vi "Filter Event Data.vi"(8 "error in (no error)":errorcluster, 10 "EventFilter Reference":T1, 11 "ControlDragStartingMsg In":refnum<class "ControlDragStartingMsg.lvclass">) -> (0 "error out":errorcluster, 2 "Discard?":bool, 3 "ControlDragStartingMsg Out":refnum<class "ControlDragStartingMsg.lvclass">)   [LabVIEW 2019, in "ActorEvents.lvlib" / "ControlDragStartingMsg.lvclass"]
uses:
  <vilib>/gpm_packages/@cs/mva-viewable/Source/ActorEvents/IEventAggregator Messages/ControlDragStartingMsg/ControlDragStartingMsg.lvclass
  <vilib>/gpm_packages/@cs/mva-viewable/Source/ActorEvents/IEventFilter/EventFilter Reference.ctl
  <vilib>/gpm_packages/@cs/mva-viewable/Source/ActorEvents/IEventFilter/IEventFilter.lvclass
  <vilib>/gpm_packages/@cs/mva-viewable/Source/ActorEvents/IEventAggregator Messages/ControlDragStartingMsg/ControlDragStartingMsg.lvclass/ControlDragStartingMsg.ctl
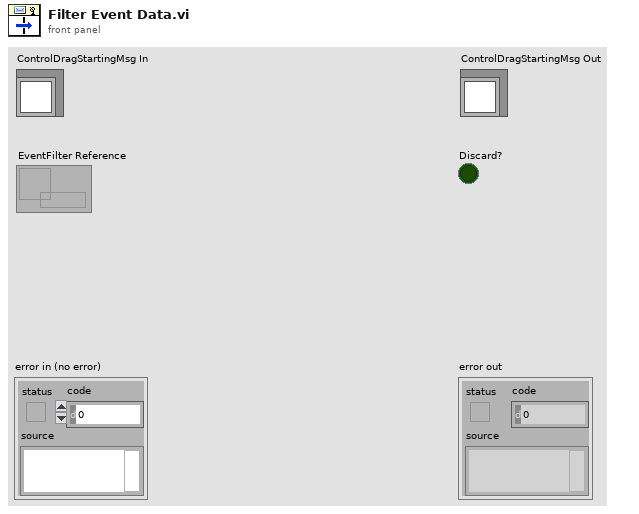
[diagram p1: front panel]
types:
  T1 = typedef "ActorEvents.lvlib/IEventFilter.lvclass/EventFilter Reference.ctl" = refnum<data-value>
  T2 = cluster{"Data":cluster{"data name":string, "drag data":variant}[], "Drag Mode":enum32{"copy or move", "copy only", "move only"}}
  T3 = cluster{"data name":string, "drag data":variant}[]
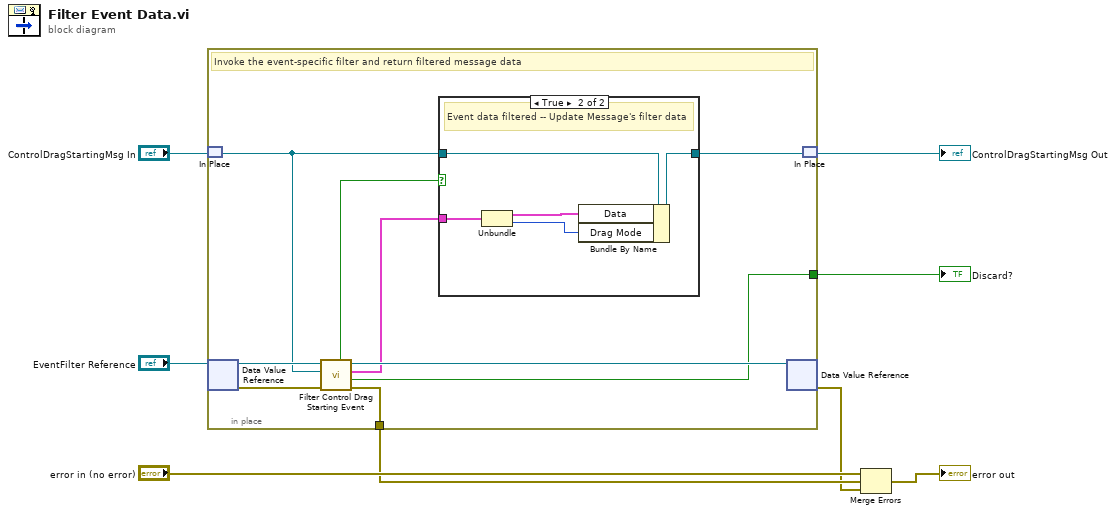
[diagram p0: block diagram]
diagram:
  n1 = in-place {
    in-place-border: [w13] -> w5
    in-place-border: [w14] -> w3
    # "Invoke the event-specific filter and return filtered message data"
    n2 = in-place-match #1("ControlDragStartingMsg In") -> (w10:refnum<class "ControlDragStartingMsg.lvclass">)
    n3 = in-place-dvr #2("EventFilter Reference") -> (w17:refnum<class "IEventFilter.lvclass">, w15:errorcluster)
    n4 = call-dynamic "Filter Control Drag Starting Event.vi"("error in (no error)"=w15, "ControlDragStartingMsg"=w10, "IEventFilter in"=w17) -> ("error out"=w13:errorcluster, "Discard?"=w14:bool, "Filtered Event Data"=w11:T2, "IEventFilter out"=w16:refnum<class "IEventFilter.lvclass">, "Data Filtered?"=w12:bool)  [unwired: 4 in]
    n5 = case shown="True" w12 {
      tunnel: w11 -> [_ w21]
      tunnel: w10 -> [w18 w23]
      tunnel: [w18 w22] -> w9
      frame False {
        # "No data filtered"
      }
      frame True {
        # "Event data filtered -- Update Message's filter data"
        n6 = Unbundle(w21) -> ("Data"=w20:T3, "Drag Mode"=w19:enum32{"copy or move", "copy only", "move only"})
        n7 = Bundle By Name(cluster=w23, "Data"=w20, "Drag Mode"=w19) -> (w22:refnum<class "ControlDragStartingMsg.lvclass">)
      }
    }
    n8 = in-place-dvr #2(w16) -> (w4:errorcluster)  [unwired: 1 out]
    n9 = in-place-match #1(w9) -> (→"ControlDragStartingMsg Out":refnum<class "ControlDragStartingMsg.lvclass">)
  }
  "Discard?" <- w3
  n10 = Merge Errors("error in (no error)", w5, w4) -> (→"error out":errorcluster)
